vi "FPGA_Vih meas with K24xx.vi"() -> ()   [LabVIEW 2010]
uses:
  Софт/Keithley 24XX/Keithley 24XX.lvlib
panel:
  in  "Begin Level, V":dbl
  out "Err Out":errorcluster
  out "Err In":errorcluster
  out "VISA In":refnum<visa-resource-name>
  out "VISA Out":refnum<visa-resource-name>
  in  "Vil, V":dbl
  in  "Vih, V":dbl
  in  "Step, V":dbl
  in  "ErrIn In":errorcluster
  in  "VISA In":refnum<visa-resource-name>
  in  "VISA Out":refnum<visa-resource-name>
  in  "MeasF Out":string
  in  "Err Out":errorcluster
  out "Vih meas, В":dbl format="%#.3g"
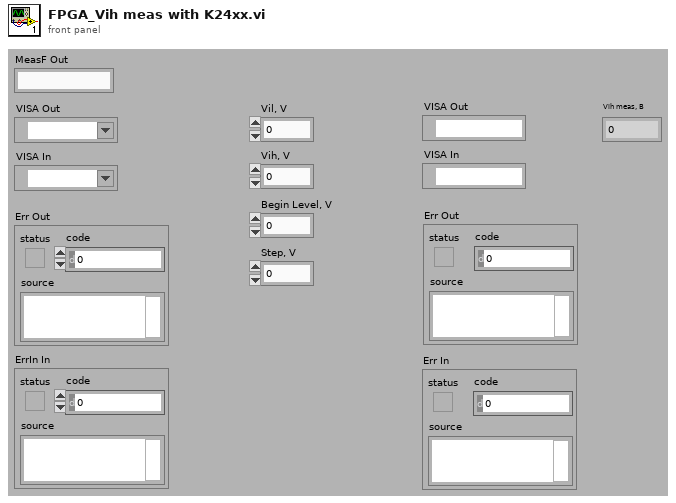
[diagram p1: front panel]
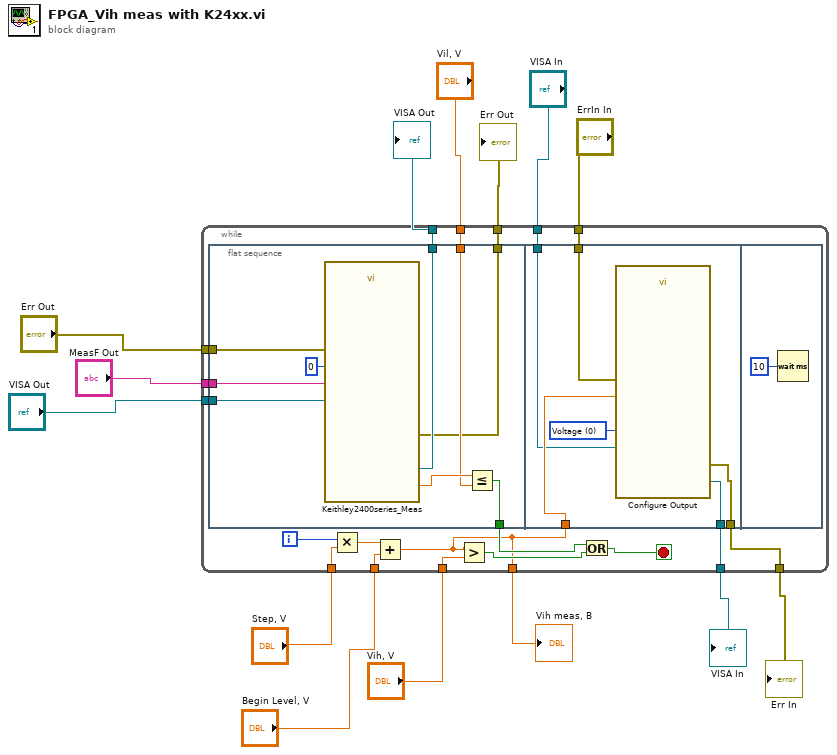
[diagram p0: block diagram]
diagram:
  n1 = while {
    tunnel: [w28] -> w8
    tunnel: "Err Out" -> [w27]
    tunnel: "MeasF Out" -> [w26]
    tunnel: "VISA Out" -> [w25]
    tunnel: "ErrIn In" -> [w24]
    tunnel: "VISA In" -> [w23]
    tunnel: "Step, V" -> [w22]
    tunnel: "Vih, V" -> [w21]
    tunnel: "Vil, V" -> [w20]
    tunnel: [w19] -> w6
    tunnel: [w18] -> w5
    tunnel: [w17] -> w4
    tunnel: [w16] -> w3
    tunnel: "Begin Level, V" -> [w15]
    i -> [w33]
    stop <- w29 stop-if-true
    n2 = flat-sequence {
      tunnel: [w41] -> w31
      tunnel: w27 -> [w39]
      tunnel: w26 -> [w38]
      tunnel: w25 -> [w37]
      tunnel: w20 -> [w36]
      tunnel: [w35] -> w19
      tunnel: [w34] -> w16
      tunnel: w28 -> [w47]
      tunnel: w24 -> [w46]
      tunnel: w23 -> [w45]
      tunnel: [w44] -> w18
      tunnel: [w43] -> w17
      frame #0 {
        n3 = call "Keithley2400series_Meas.vi"("MEAS:<f>"=w38, "error in (no error)"=w39, "MEAS mode, 0 Volt"=u16 0, "VISA resource name in"=w37) -> ("error out"=w34:errorcluster, "Замер"=w42:dbl, "VISA out"=w35:refnum<visa-resource-name>)  [unwired: 1 in, 1 out]
        n4 = Less Or Equal?(x=w42, y=w36) -> (x <= y?=w41:bool)
      }
      frame #1 {
        w48 = u16 0 items=["Voltage", "Current"] ("Source Mode  (0: Voltage)")
        n5 = call "Configure Output.vi"("Source Mode  (0: Voltage)"=w48, "error in (no error)"=w46, "Output Level (0)"=w47, "VISA resource name"=w45) -> ("error out"=w43:errorcluster, "VISA resource name out"=w44:refnum<visa-resource-name>)  [unwired: 6 in]
      }
      frame #2 {
        n6 = Wait (ms)(milliseconds to wait=u32 10) -> ()  [unwired: 1 out]
      }
    }
    n7 = Multiply(x=w33, y=w22) -> (x*y=w32:dbl)
    n8 = Add(x=w32, y=w15) -> (x+y=w28:dbl)
    n9 = Greater?(x=w28, y=w21) -> (0:w30:bool)
    n10 = Or(x=w31, y=w30) -> (x .or. y?=w29:bool)
  }
  "Vih meas, В" <- w8
  "VISA Out" <- w6
  "VISA In" <- w5
  "Err In" <- w4
  "Err Out" <- w3
